vi "APC_9056_NGControl.vi"(1 "LoadIni?":bool, 2 "PC_ControlSettings":T2={"Spark advance [CADBTDC]"=0.0, "Pref"=0.0, "O2ref"=0.0, "DI advance [CADBTDC]"=0.0, "DI duration [ms] "=0.0, "CO2ref"=0.0, "PFI duration [ms]"=0.0, "IMEP ref"=0.0, "Speed ref"=0.0, "IGN enable"=TRUE, "DI enable"=TRUE, "CL PFI\n lambda"=TRUE, "CL PFI\nIMEP"=FALSE, "Activate\ncylinder"=[FALSE, FALSE, FALSE, FALSE, FALSE, FALSE], "Force idling"=FALSE, "Force motoring"=FALSE, "ETP resync"=FALSE, "Requested mode"=0, "Clear Sync Errors"=FALSE, "toggle TDC"=FALSE, "l ref"=0.0, "PID control references"={"NG"=FALSE, "Ar"=FALSE, "O2"=FALSE, "Intake vent"=FALSE, "Cross vent"=FALSE, "Exhaust vent"=FALSE, "NG control mode"=0, "NG-FC-001-REF"=0.0, "WF-OA-002-REF"=0.0, "IMEP-REF"=0.0, "Nm-REF"=0.0, "Ar control mode"=0, "AR-PC-002-REF"=0.0, "WF-PT-004-REF"=0.0, "O2 control mode"=0, "O2-FC-001-REF"=0.0, "WF-OA-001-REF"=0.0, "Tcoolant control  mode"=0, "EC-FC-001-REF"=0.0, "EC-TT-001-REF"=0.0, "Texh control mode"=0, "SW-FC-004-REF"=0.0, "SW-FT-002-REF"=0.0, "WF-TT-004-REF"=0.0, "Toil control mode"=0, "SW-FC-009-REF"=0.0, "SW-FT-004-REF"=0.0, "EO-TT-001-REF"=0.0, "AIC201_CO2_ConcTarget"=0.0, "O2_FF_NG"=FALSE, "Dyno control mode"=0, "Membrane control mode"=0, "AR-FT-001-REF"=0.0, "MTR modbus floats"=[0.0, 0.0, 0.0, 0.0, 0.0, 0.0, 0.0, 0.0, 0.0, 0.0, 0.0, 0.0, 0.0, 0.0, 0.0, 0.0, 0.0, 0.0, 0.0], "MTR modbus u16"=[0, 0, 0, 0, 0, 0, 0], "MTR HB"=FALSE, "PC_HB"=FALSE, "EMERGENCY STOP"=FALSE}, "CA50setpoint [CADATDC]"=0.0, "CA50 control"=TRUE, "Knock control"=TRUE, "CLEAR EMERGENCY STOP"=FALSE, "EMERGENCY STOP"=FALSE}, 3 "input cluster":T4) -> (0 "NG-FC-001-REF":dbl format="%.2f")   [LabVIEW 2020]
uses:
  controls/APC_PIDCluster.ctl
  controls/APC_ControlSettings.ctl
  controls/APC_PIDcontrolSettings.ctl
  controls/APC_NG_PIDsettings.ctl
  <vilib>/addons/control/pid/pid.llb/PID Advanced (DBL).vi
  <vilib>/Utility/xml.llb/Write to XML File(string).vi
  <vilib>/Utility/xml.llb/Read From XML File(string).vi
  <vilib>/addons/control/pid/NI_PID_pid.lvlib
panel:
  out "direct?":bool
  out "inv(lambda)":dbl
  out "Lambda":dbl
  out "IMEPn6":dbl
  out "TORQUE":dbl
  in  "FF control IMEP":dbl format="%.2f"
  in  "PID gains IMEP":T1={"proportional gain (Kc)"=1.0, "integral time (Ti, min)"=0.01, "derivative time (Td, min)"=0.0} {"derivative time (Td, min)" format="%.3f"; "integral time (Ti, min)" format="%.3f"; "proportional gain (Kc)" format="%.3f"}
  in  "PID setpoint range IMEP":cluster{"setpoint high":dbl, "setpoint low":dbl}={"setpoint high"=100.0, "setpoint low"=0.0} {"setpoint high" format="%.2f"; "setpoint low" format="%.2f"}
  in  "FF control TORQUE":dbl format="%.2f"
  in  "PID gains TORQUE":T1={"proportional gain (Kc)"=1.0, "integral time (Ti, min)"=0.01, "derivative time (Td, min)"=0.0} {"derivative time (Td, min)" format="%.3f"; "integral time (Ti, min)" format="%.3f"; "proportional gain (Kc)" format="%.3f"}
  in  "PID setpoint range TORQUE":cluster{"setpoint high":dbl, "setpoint low":dbl}={"setpoint high"=100.0, "setpoint low"=0.0} {"setpoint high" format="%.2f"; "setpoint low" format="%.2f"}
  out "SAFE":bool
  out "NG-FC-001":dbl
  in  "NG-FC-001-REF (manual)":dbl
  in  "TORQUE-REF (manual)":dbl
  in  "save":bool
  in  "load":bool
  out "Process point":dbl
  in  "IMEP-REF (manual)":dbl
  in  "WF-OA-002-Lambda-REF (manual)":dbl
  in  "NG control mode (manual)":u8
  out "CL on?":bool
  out "CL setpoint":dbl format="%.2f"
  in  "Override PC PID references":bool
  in  "learn?":bool
  in  "FF control LAMBDA":dbl format="%.2f"
  in  "PID gains LAMBDA":T1={"proportional gain (Kc)"=1.0, "integral time (Ti, min)"=0.01, "derivative time (Td, min)"=0.0} {"derivative time (Td, min)" format="%.3f"; "integral time (Ti, min)" format="%.3f"; "proportional gain (Kc)" format="%.3f"}
  in  "PID setpoint range inv(LAMBDA)":cluster{"setpoint high":dbl, "setpoint low":dbl}={"setpoint high"=100.0, "setpoint low"=0.0} {"setpoint high" format="%.2f"; "setpoint low" format="%.2f"}
  in  "PID output range":cluster{"output high":dbl, "output low":dbl}={"output high"=100.0, "output low"=-100.0} {"output low" format="%.2f"; "output high" format="%.2f"}
  in  "Safe mode control":dbl format="%.2f"
  in  "reinitialize ?":bool
  out "Direct control":dbl format="%.2f"
  # "NG CONTROL MODES\n0.- safe mode\n1.- manual\n2.- closed loop control: modes 4, 5 and 6 used for selecting the feedback variable (lambda, IMEP or torque). Mode 2 is default (lambda)\nFor the case of lambda, inverse is later applied"
  # "NG control"
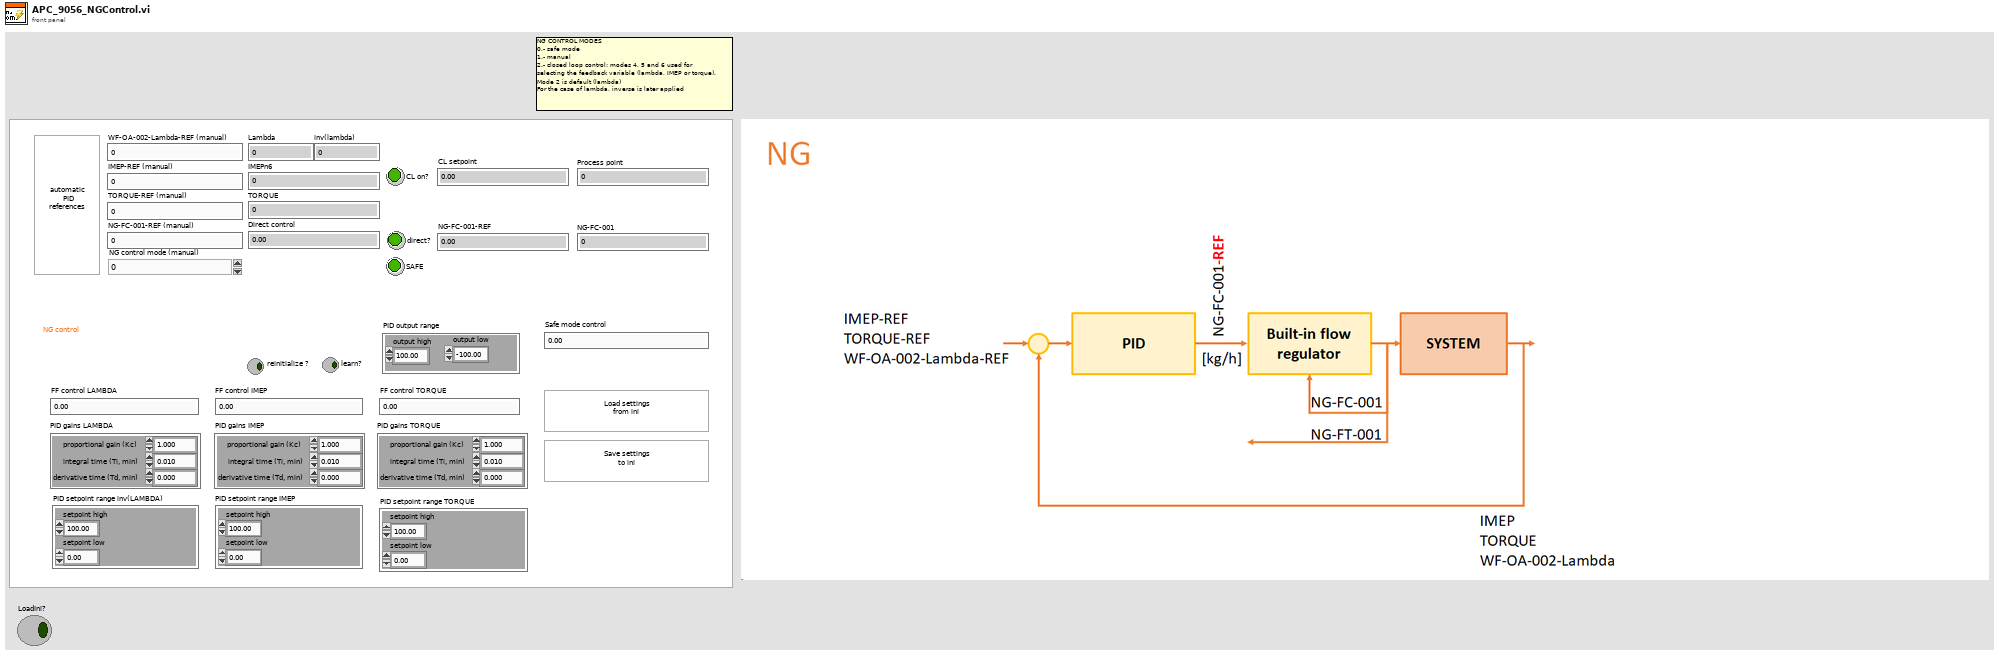
[diagram p1: front panel]
types:
  T1 = cluster{"proportional gain (Kc)":dbl, "integral time (Ti, min)":dbl, "derivative time (Td, min)":dbl}
  T2 = typedef "APC_ControlSettings.ctl" = cluster{"Spark advance [CADBTDC]":dbl, "Pref":dbl, "O2ref":dbl, "DI advance [CADBTDC]":dbl, "DI duration [ms] ":dbl, "CO2ref":dbl, "PFI duration [ms]":dbl, "IMEP ref":dbl, "Speed ref":dbl, "IGN enable":bool, "DI enable":bool, "CL PFI\n lambda":bool, "CL PFI\nIMEP":bool, "Activate\ncylinder":bool[], "Force idling":bool, "Force motoring":bool, "ETP resync":bool, "Requested mode":i8, "Clear Sync Errors":bool, "toggle TDC":bool, "l ref":dbl, "PID control references":T3, "CA50setpoint [CADATDC]":dbl, "CA50 control":bool, "Knock control":bool, "CLEAR EMERGENCY STOP":bool, "EMERGENCY STOP":bool}
  T3 = typedef "APC_PIDcontrolSettings.ctl" = cluster{"NG":bool, "Ar":bool, "O2":bool, "Intake vent":bool, "Cross vent":bool, "Exhaust vent":bool, "NG control mode":u8, "NG-FC-001-REF":dbl, "WF-OA-002-REF":dbl, "IMEP-REF":dbl, "Nm-REF":dbl, "Ar control mode":u8, "AR-PC-002-REF":dbl, "WF-PT-004-REF":dbl, "O2 control mode":u8, "O2-FC-001-REF":dbl, "WF-OA-001-REF":dbl, "Tcoolant control  mode":u8, "EC-FC-001-REF":dbl, "EC-TT-001-REF":dbl, "Texh control mode":u8, "SW-FC-004-REF":dbl, "SW-FT-002-REF":dbl, "WF-TT-004-REF":dbl, "Toil control mode":u8, "SW-FC-009-REF":dbl, "SW-FT-004-REF":dbl, "EO-TT-001-REF":dbl, "AIC201_CO2_ConcTarget":dbl, "O2_FF_NG":bool, "Dyno control mode":u8, "Membrane control mode":u8, "AR-FT-001-REF":dbl, "MTR modbus floats":sgl[], "MTR modbus u16":u16[], "MTR HB":bool, "PC_HB":bool, "EMERGENCY STOP":bool}
  T4 = typedef "APC_PIDCluster.ctl" = cluster{"AR-FT-001":dbl, "O2-FC-001":dbl, "SW-FT-004":dbl, "SW-FT-002":dbl, "WF-OA-002":dbl, "WF-PT-004":dbl, "WF-OA-001":dbl, "EC-TT-001":dbl, "WF-TT-004":dbl, "EC-FC-001":dbl, "NG-FC-001":dbl, "EO-TT-001":dbl, "SW-FC-008":dbl, "SW-FC-004":dbl, "IMEPn6":dbl, "TORQUE":dbl, "CylPresWarnings":dbl, "CylPresErrors":dbl, "NG-FT-001":dbl, "EngineSpeed_rpm":dbl}
  T5 = typedef "APC_NG_PIDsettings.ctl" = cluster{"PID output range":cluster{"output high":dbl, "output low":dbl}, "FF control LAMBDA":dbl, "PID gains LAMBDA":cluster{"proportional gain (Kc)":dbl, "integral time (Ti, min)":dbl, "derivative time (Td, min)":dbl}, "PID setpoint range inv(LAMBDA)":cluster{"setpoint high":dbl, "setpoint low":dbl}, "FF control IMEP":dbl, "PID gains IMEP":cluster{"proportional gain (Kc)":dbl, "integral time (Ti, min)":dbl, "derivative time (Td, min)":dbl}, "PID setpoint range IMEP":cluster{"setpoint high":dbl, "setpoint low":dbl}, "FF control TORQUE":dbl, "PID gains TORQUE":cluster{"proportional gain (Kc)":dbl, "integral time (Ti, min)":dbl, "derivative time (Td, min)":dbl}, "PID setpoint range TORQUE":cluster{"setpoint high":dbl, "setpoint low":dbl}, "Safe mode control":dbl}
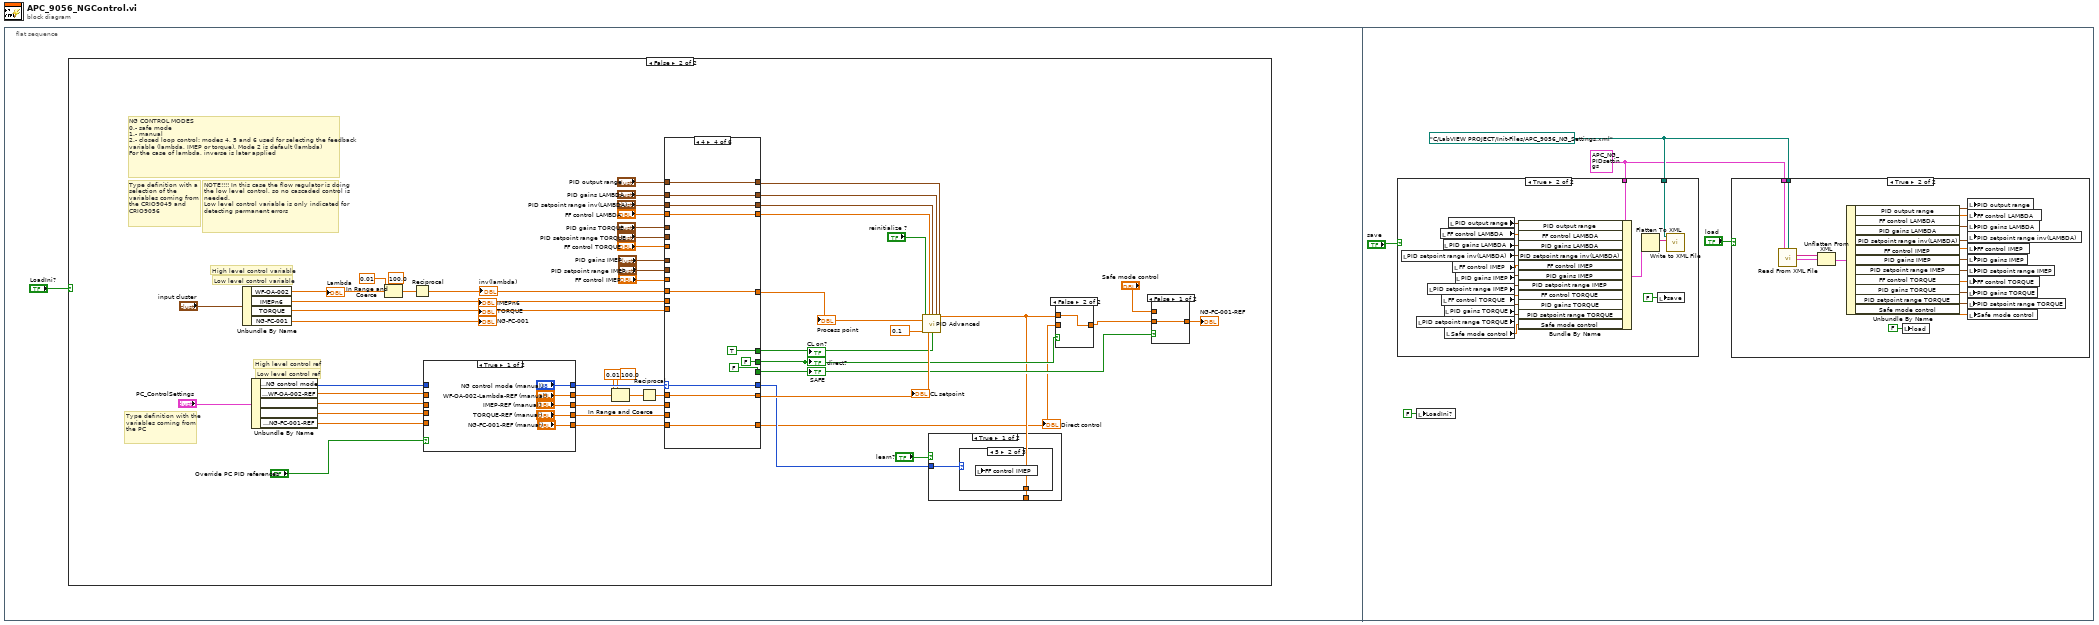
[diagram p0: block diagram]
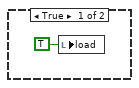
[diagram p2: hidden frame]
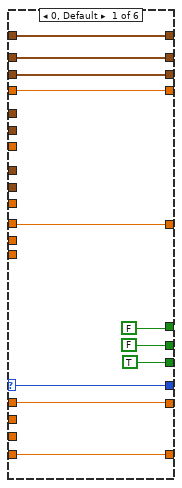
[diagram p4: hidden frame]
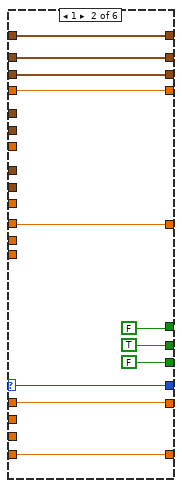
[diagram p5: hidden frame]
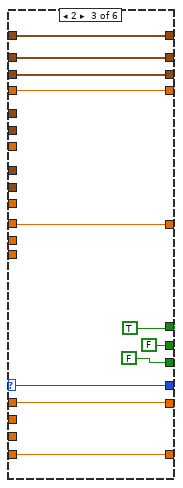
[diagram p6: hidden frame]
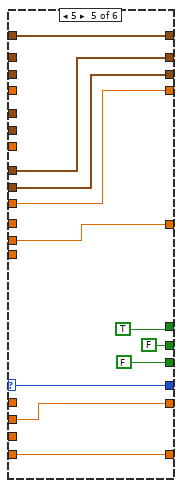
[diagram p7: hidden frame]
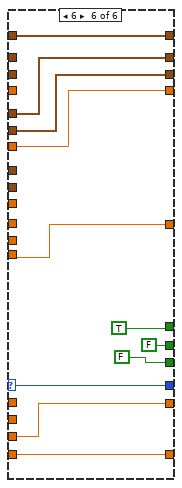
[diagram p8: hidden frame]
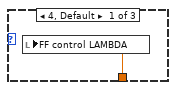
[diagram p10: hidden frame]
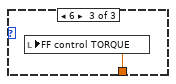
[diagram p11: hidden frame]
diagram:
  n1 = flat-sequence {
    frame #0 {
      n2 = case shown="False" "LoadIni?" {
        frame True {
          n3 = local write "load"(TRUE ("load")) -> ()
        }
        frame False {
          # "NOTE!!!! In this case the flow regulator is doing the low level control, so no cascaded control is needed.\nLow level control variable is only indicated for detecting permanent errors"
          # "Type definition with a selection of the variables coming from the CRIO9049 and CRIO9056"
          # "Type definition with the variables coming from the PC"
          # "Low level control ref"
          # "Low level control variable"
          # "High level control ref"
          # "High level control variable"
          # "NG CONTROL MODES\n0.- safe mode\n1.- manual\n2.- closed loop control: modes 4, 5 and 6 used for selecting the feedback variable (lambda, IMEP or torque). Mode 2 is default (lambda)\nFor the case of lambda, inverse is later applied"
          n4 = Unbundle By Name("input cluster") -> ("WF-OA-002"=w17:dbl, "IMEPn6"=w46:dbl, "TORQUE"=w45:dbl, "NG-FC-001"=→"NG-FC-001":dbl)
          "TORQUE" <- w45
          "IMEPn6" <- w46
          "Lambda" <- w17
          n5 = Unbundle By Name("PC_ControlSettings") -> ("PID control references.NG control mode"=w48:u8, "PID control references.WF-OA-002-REF"=w44:dbl, "PID control references.IMEP-REF"=w43:dbl, "PID control references.Nm-REF"=w42:dbl, "PID control references.NG-FC-001-REF"=w41:dbl)
          n6 = In Range and Coerce(upper limit=100.0, x=w17, lower limit=0.01) -> (coerced(x)=w16:dbl)  [unwired: 1 out]
          n7 = Reciprocal(x=w16) -> (1/x=w18:dbl)
          "inv(lambda)" <- w18
          n8 = case shown="True" "Override PC PID references" {
            tunnel: w48 -> [_ w140]
            tunnel: w44 -> [_ w139]
            tunnel: w43 -> [_ w138]
            tunnel: ["NG control mode (manual)" w140] -> w37
            tunnel: ["WF-OA-002-Lambda-REF (manual)" w139] -> w10
            tunnel: ["IMEP-REF (manual)" w138] -> w39
            tunnel: w42 -> [_ w137]
            tunnel: w41 -> [_ w136]
            tunnel: ["TORQUE-REF (manual)" w137] -> w36
            tunnel: ["NG-FC-001-REF (manual)" w136] -> w40
            frame True {
            }
            frame False {
            }
          }
          n9 = In Range and Coerce(upper limit=100.0, x=w10, lower limit=0.01) -> (coerced(x)=w13:dbl)  [unwired: 1 out]
          n10 = Reciprocal(x=w13) -> (1/x=w9:dbl)
          n11 = case shown="4" w37 {
            selector: w37 -> [w66 w77 w87 w99 w110 w120]
            tunnel: w45 -> [_ _ _ _ _ w123]
            tunnel: w46 -> [_ _ _ _ w112 _]
            tunnel: w18 -> [w68 w79 w90 w101 _ _]
            tunnel: [w68 w79 w90 w101 w112 w123] -> w8
            tunnel: w9 -> [w67 w78 w89 w98 _ _]
            tunnel: w39 -> [_ _ _ _ w111 _]
            tunnel: [w67 w78 w89 w98 w111 w122] -> w38
            tunnel: w40 -> [w65 w76 w88 w100 w109 w121]
            tunnel: [w65 w76 w88 w100 w109 w121] -> w3
            tunnel: [w66 w77 w87 w99 w110 w120] -> w20
            tunnel: w36 -> [_ _ _ _ _ w122]
            tunnel: [FALSE ("auto? (T)") FALSE ("auto? (T)") TRUE ("auto? (T)") TRUE ("auto? (T)") TRUE ("auto? (T)") TRUE ("auto? (T)")] -> w35
            tunnel: [TRUE ("auto? (T)") FALSE ("auto? (T)") FALSE ("auto? (T)") FALSE ("auto? (T)") FALSE ("auto? (T)") FALSE ("auto? (T)")] -> w19
            tunnel: [w62 w73 w84 w92 w106 w117] -> w34
            tunnel: "PID output range" -> [w62 w73 w84 w92 w106 w117]
            tunnel: "PID gains LAMBDA" -> [w61 w72 w83 w95 _ _]
            tunnel: "PID setpoint range inv(LAMBDA)" -> [w60 w71 w82 w94 _ _]
            tunnel: "FF control LAMBDA" -> [w59 w70 w81 w93 _ _]
            tunnel: [w61 w72 w83 w95 w105 w116] -> w29
            tunnel: [w60 w71 w82 w94 w104 w115] -> w28
            tunnel: [w59 w70 w81 w93 w103 w114] -> w7
            tunnel: "PID gains TORQUE" -> [_ _ _ _ _ w116]
            tunnel: "PID setpoint range TORQUE" -> [_ _ _ _ _ w115]
            tunnel: "FF control TORQUE" -> [_ _ _ _ _ w114]
            tunnel: "PID gains IMEP" -> [_ _ _ _ w105 _]
            tunnel: "PID setpoint range IMEP" -> [_ _ _ _ w104 _]
            tunnel: "FF control IMEP" -> [_ _ _ _ w103 _]
            tunnel: [FALSE ("auto? (T)") TRUE ("auto? (T)") FALSE ("auto? (T)") FALSE ("auto? (T)") FALSE ("auto? (T)") FALSE ("auto? (T)")] -> w6
            frame 0, Default {
            }
            frame 1 {
            }
            frame 2 {
            }
            frame 4 {
            }
            frame 5 {
            }
            frame 6 {
            }
          }
          "Direct control" <- w3
          "CL setpoint" <- w38
          "CL on?" <- w35
          "Process point" <- w8
          "SAFE" <- w19
          "direct?" <- w6
          n12 = call-poly <vilib>:"PID Advanced.vi"("setpoint"=w38, "output range"=w34, "auto? (T)"=w35, "manual control"=w7, "process variable"=w8, "setpoint range"=w28, "PID gains"=w29, "dt (s)"=0.1, "reinitialize? (F)"="reinitialize ?") -> ("output"=w5:dbl)  [unwired: 5 in, 1 out]
          n13 = case shown="True" "learn?" {
            tunnel: w5 -> [w127 _]
            tunnel: w20 -> [w126 _]
            frame True {
              n14 = case shown="5" w126 {
                tunnel: w127 -> [w128 w129 w130]
                frame 4, Default {
                  n15 = local write "FF control LAMBDA"(w128) -> ()
                }
                frame 5 {
                  n16 = local write "FF control IMEP"(w129) -> ()
                }
                frame 6 {
                  n17 = local write "FF control TORQUE"(w130) -> ()
                }
              }
            }
            frame False {
            }
          }
          n18 = case shown="False" w6 {
            tunnel: [w56 w57] -> w4
            tunnel: w5 -> [_ w57]
            tunnel: w3 -> [w56 _]
            frame True {
            }
            frame False {
            }
          }
          n19 = case shown="False" w19 {
            tunnel: [w124 w125] -> w51
            tunnel: "Safe mode control" -> [_ w125]
            tunnel: w4 -> [w124 _]
            frame False {
            }
            frame True {
            }
          }
          "NG-FC-001-REF" <- w51
        }
      }
    }
    frame #1 {
      w142 = T5 {"PID output range"={"output high"=100.0, "output low"=-100.0}, "FF control LAMBDA"=0.0, "PID gains LAMBDA"={"proportional gain (Kc)"=1.0, "integral time (Ti, min)"=0.01, "derivative time (Td, min)"=0.0}, "PID setpoint range inv(LAMBDA)"={"setpoint high"=100.0, "setpoint low"=0.0}, "FF control IMEP"=0.0, "PID gains IMEP"={"proportional gain (Kc)"=1.0, "integral time (Ti, min)"=0.01, "derivative time (Td, min)"=0.0}, "PID setpoint range IMEP"={"setpoint high"=100.0, "setpoint low"=0.0}, "FF control TORQUE"=0.0, "PID gains TORQUE"={"proportional gain (Kc)"=1.0, "integral time (Ti, min)"=0.01, "derivative time (Td, min)"=0.0}, "PID setpoint range TORQUE"={"setpoint high"=100.0, "setpoint low"=0.0}, "Safe mode control"=0.0} ("NG PID settings")
      w143 = path "C:/LabVIEW PROJECT/Init-Files/APC_9056_NG_Settings.xml" ("XML File Path")
      n20 = case shown="True" "save" {
        tunnel: w143 -> [_ w175]
        tunnel: w142 -> [_ w174]
        frame False {
        }
        frame True {
          n21 = local read "PID setpoint range inv(LAMBDA)"() -> (w169:cluster{"setpoint high":dbl, "setpoint low":dbl})
          n22 = local read "PID setpoint range TORQUE"() -> (w163:cluster{"setpoint high":dbl, "setpoint low":dbl})
          n23 = local read "PID setpoint range IMEP"() -> (w166:cluster{"setpoint high":dbl, "setpoint low":dbl})
          n24 = local read "FF control LAMBDA"() -> (w171:dbl)
          n25 = local read "FF control TORQUE"() -> (w165:dbl)
          n26 = local read "PID gains LAMBDA"() -> (w170:T1)
          n27 = local read "PID gains TORQUE"() -> (w164:T1)
          n28 = local read "Safe mode control"() -> (w162:dbl)
          n29 = local read "PID output range"() -> (w172:cluster{"output high":dbl, "output low":dbl})
          n30 = local read "FF control IMEP"() -> (w168:dbl)
          n31 = local read "PID gains IMEP"() -> (w167:T1)
          n32 = Bundle By Name(cluster=w174, "PID output range"=w172, "FF control LAMBDA"=w171, "PID gains LAMBDA"=w170, "PID setpoint range inv(LAMBDA)"=w169, "FF control IMEP"=w168, "PID gains IMEP"=w167, "PID setpoint range IMEP"=w166, "FF control TORQUE"=w165, "PID gains TORQUE"=w164, "PID setpoint range TORQUE"=w163, "Safe mode control"=w162) -> (w177:T5)
          n33 = Flatten To XML(6:w177) -> (2:w176:string)
          n34 = local write "save"(FALSE ("load")) -> ()
          n35 = call-poly <vilib>:"Write to XML File.vi"("XML Input"=w176, "XML File Path"=w175) -> ()  [unwired: 7 in, 3 out]
        }
      }
      n36 = local write "LoadIni?"(FALSE ("LoadIni?")) -> ()
      n37 = case shown="True" "load" {
        tunnel: w143 -> [_ w160]
        tunnel: w142 -> [_ w159]
        frame False {
        }
        frame True {
          n38 = call-poly <vilib>:"Read From XML File.vi"("XML File Path"=w160) -> ("XML Elements"=w161:string)  [unwired: 8 in, 2 out]
          n39 = Unflatten From XML(xml string=w161, type=w159) -> (value=w158:T5)  [unwired: 1 in, 1 out]
          n40 = Unbundle By Name(w158) -> ("PID output range"=w156:cluster{"output high":dbl, "output low":dbl}, "FF control LAMBDA"=w155:dbl, "PID gains LAMBDA"=w154:T1, "PID setpoint range inv(LAMBDA)"=w153:cluster{"setpoint high":dbl, "setpoint low":dbl}, "FF control IMEP"=w152:dbl, "PID gains IMEP"=w151:T1, "PID setpoint range IMEP"=w150:cluster{"setpoint high":dbl, "setpoint low":dbl}, "FF control TORQUE"=w149:dbl, "PID gains TORQUE"=w148:T1, "PID setpoint range TORQUE"=w147:cluster{"setpoint high":dbl, "setpoint low":dbl}, "Safe mode control"=w146:dbl)
          n41 = local write "load"(FALSE ("save")) -> ()
          n42 = local write "FF control TORQUE"(w149) -> ()
          n43 = local write "PID gains TORQUE"(w148) -> ()
          n44 = local write "PID setpoint range TORQUE"(w147) -> ()
          n45 = local write "PID output range"(w156) -> ()
          n46 = local write "FF control LAMBDA"(w155) -> ()
          n47 = local write "PID gains LAMBDA"(w154) -> ()
          n48 = local write "PID setpoint range inv(LAMBDA)"(w153) -> ()
          n49 = local write "FF control IMEP"(w152) -> ()
          n50 = local write "PID gains IMEP"(w151) -> ()
          n51 = local write "PID setpoint range IMEP"(w150) -> ()
          n52 = local write "Safe mode control"(w146) -> ()
        }
      }
    }
  }
